vi "Write VISA resource name.vi"(8 "error in (no error)":errorcluster, 10 "VISA resource name":refnum<visa-resource-name>, 11 "Mag Lab Hardware in":refnum<class "Mag Lab Hardware.lvclass">) -> (0 "error out":errorcluster, 3 "Mag Lab Hardware out":refnum<class "Mag Lab Hardware.lvclass">)   [LabVIEW 2015, in "Mag Lab Hardware.lvclass"]
uses:
  Mag Lab Hardware.lvclass
  Mag Lab Hardware.lvclass/Mag Lab Hardware.ctl
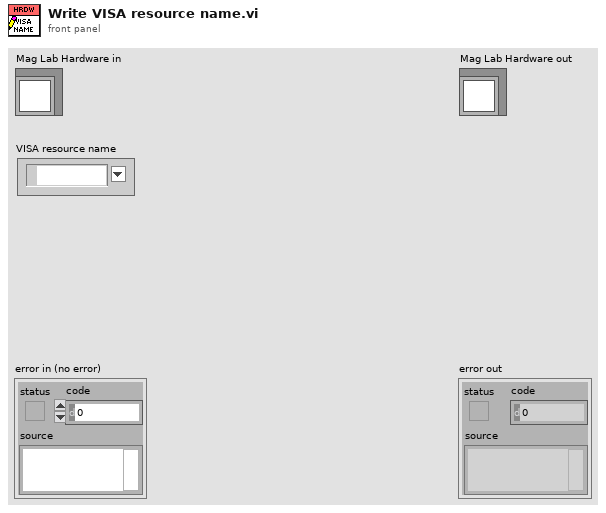
[diagram p1: front panel]
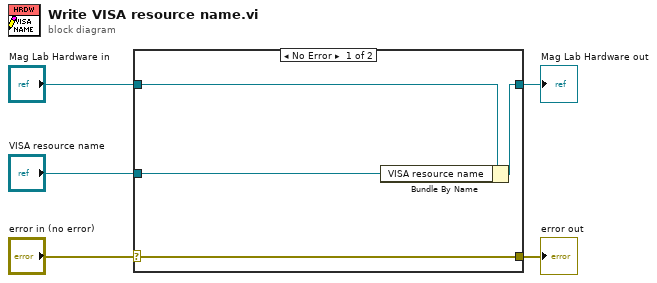
[diagram p0: block diagram]
diagram:
  n1 = case shown="No Error" "error in (no error)" {
    selector: "error in (no error)" -> [w9 w10]
    tunnel: [w9 w10] -> w4
    tunnel: [w7 w11] -> w2
    tunnel: "Mag Lab Hardware in" -> [w8 w11]
    tunnel: "VISA resource name" -> [w6 _]
    frame No Error {
      n2 = Bundle By Name(cluster=w8, "VISA resource name"=w6) -> (w7:refnum<class "Mag Lab Hardware.lvclass">)
    }
    frame Error {
    }
  }
  "error out" <- w4
  "Mag Lab Hardware out" <- w2
